vi "read_heater_spinner.vi"() -> (7 "Heater/Spinner Remote":bool, 8 "Spinner":bool, 9 "Heater":bool)   [LabVIEW 2011]
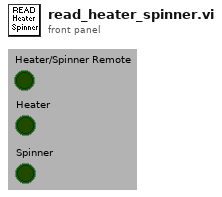
[diagram p1: front panel]
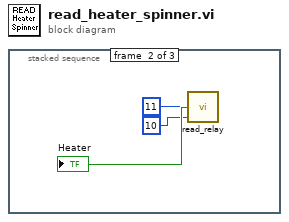
[diagram p0: block diagram]
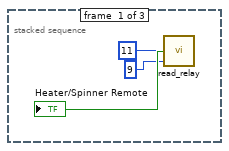
[diagram p2: hidden frame]
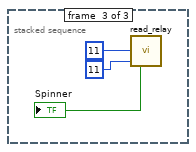
[diagram p3: hidden frame]
diagram:
  n1 = stacked-sequence {
    frame #0 {
      n2 = call "read_relay.vi"("Relay"=9, "Slot"=11) -> ("Relay Status"=→"Heater/Spinner Remote":bool)  [unwired: 1 out]
    }
    frame #1 {
      n3 = call "read_relay.vi"("Relay"=10, "Slot"=11) -> ("Relay Status"=→"Heater":bool)  [unwired: 1 out]
    }
    frame #2 {
      n4 = call "read_relay.vi"("Relay"=11, "Slot"=11) -> ("Relay Status"=→"Spinner":bool)  [unwired: 1 out]
    }
  }
